vi "Is Channel Enabled.vi"(8 "error in (no error)":errorcluster, 10 "Channel (0: Channel 1)":u16(ring) items=["Channel 1", "Channel 2", "Channel 3", "Channel 4", "Math", "Reference 1", "Reference 2", "Reference 3", "Reference 4", "Normal", "Average", "Amplitude", "Frequency", "Minimum Peak Hold", "Maximum Peak Hold", "Phase"], 11 "VISA resource name":refnum<visa-resource-name>) -> (0 "error out":errorcluster, 2 "Enabled":bool, 3 "VISA resource name out":refnum<visa-resource-name>)   [LabVIEW 2009, in "Tektronix DPO MSO 2000 4000 Series.lvlib"]
doc: "Queries whether the specified input channel is enabled to acquire a waveform from the oscilloscope."
uses:
  <instrlib>/Tektronix DPO MSO 2000 4000 Series/Tektronix DPO MSO 2000 4000 Series.lvlib
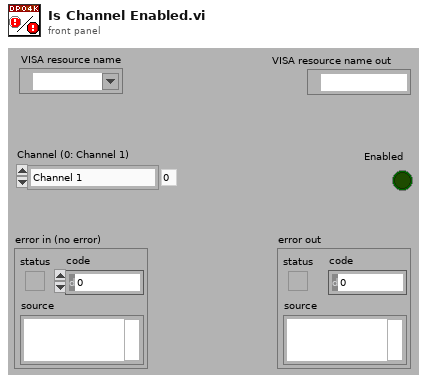
[diagram p1: front panel]
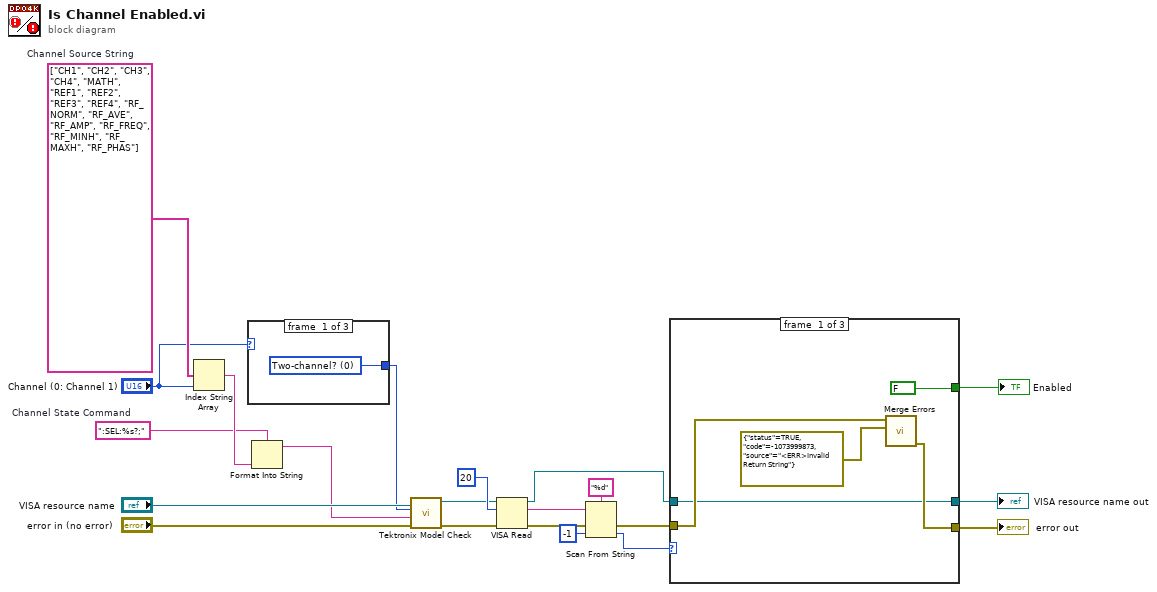
[diagram p0: block diagram]
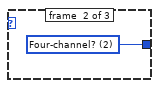
[diagram p2: hidden frame]
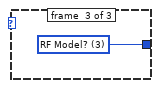
[diagram p3: hidden frame]
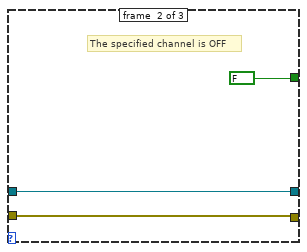
[diagram p4: hidden frame]
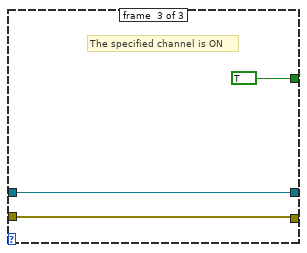
[diagram p5: hidden frame]
diagram:
  w10 = ":SEL:%s?;"  # Channel State Command
  w9 = string[] ["CH1", "CH2", "CH3", "CH4", "MATH", "REF1", "REF2", "REF3", "REF4", "RF_NORM", "RF_AVE", "RF_AMP", "RF_FREQ", "RF_MINH", "RF_MAXH", "RF_PHAS"]  # Channel Source String
  n1 = Index String Array(1:"Channel (0: Channel 1)", 2:w9) -> (0:w11:string)  [unwired: 1 in]
  n2 = case shown="0, 1, 4..8, Default" "Channel (0: Channel 1)" {
    tunnel: [w22 w23 w24] -> w4
    frame #0 {
      w22 = u16 0 items=["Two-channel?", "Digital Model?", "Four-channel?", "RF Model?"] ("Oscilloscope Model Tests (3: RF Model?)")
    }
    frame #1 {
      w23 = u16 2 items=["Two-channel?", "Digital Model?", "Four-channel?", "RF Model?"] ("Oscilloscope Model Tests (3: RF Model?)")
    }
    frame #2 {
      w24 = u16 3 items=["Two-channel?", "Digital Model?", "Four-channel?", "RF Model?"] ("Oscilloscope Model Tests (3: RF Model?)")
    }
  }
  n3 = Format Into String(format string=w10, w11) -> (resulting string=w3:string)  [unwired: 2 in, 1 out]
  n4 = call <instrlib>:"Tektronix Model Check.vi"("error in (no error)"="error in (no error)", "Command String"=w3, "Oscilloscope Model Tests (3: RF Model?)"=w4, "VISA resource name"="VISA resource name") -> ("error out"=w1:errorcluster, "VISA resource name out"=w2:refnum<visa-resource-name>)  [unwired: 6 in]
  n5 = VISA Read(VISA resource name=w2, byte count=u32 20, error in (no error)=w1) -> (VISA resource name out=w19:refnum<visa-resource-name>, read buffer=w15:string, error out=w16:errorcluster)  [unwired: 1 out]
  n6 = Scan From String(format string="%d", input string=w15, error in=w16, default 1=-1 ("default value 1")) -> (error out=w18:errorcluster, output 1=w21:i32)  [unwired: 1 in, 2 out]
  n7 = case shown="-1, Default" w21 {
    tunnel: w19 -> [w26 w32 w35]
    tunnel: w18 -> [w28 w31 w33]
    tunnel: [w27 w31 w33] -> w14
    tunnel: [w26 w32 w35] -> w13
    tunnel: [FALSE FALSE TRUE] -> w8
    frame #0 {
      n8 = call <vilib>:"Merge Errors.vi"("error in 2 (no error)"=errorcluster {"status"=TRUE, "code"=-1073999873, "source"="<ERR>Invalid Return String"} ("error out"), "error in 1 (no error)"=w28) -> ("error out"=w27:errorcluster)  [unwired: 5 in]
    }
    frame #1 {
      # "The specified channel is OFF"
    }
    frame #2 {
      # "The specified channel is ON"
    }
  }
  "error out" <- w14
  "VISA resource name out" <- w13
  "Enabled" <- w8
